vi "Append New Page.vi"(6 "Set as active (T)":bool=TRUE, 8 "error in (no error)":errorcluster, 10 "Page Name":string, 11 "Document in":refnum<class "Document.lvclass">) -> (0 "error out":errorcluster, 1 "Created?":bool, 2 "Created Page Name":string, 3 "Document out":refnum<class "Document.lvclass">)   [LabVIEW 2017, in "LabVIEW NPOI.lvlib" / "Document.lvclass"]
doc: "Create new page to the <b>Document</b>, nammed <b>Page Name</b>."
uses:
  Document.lvclass
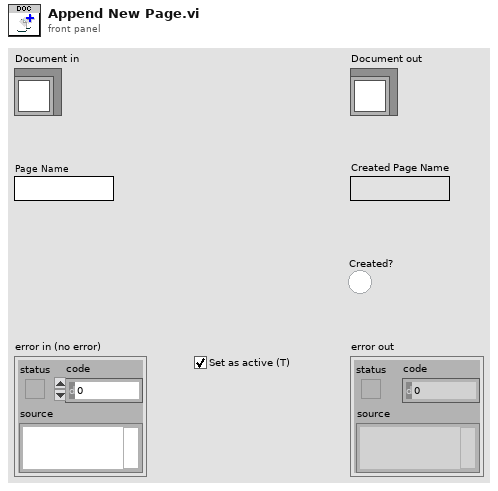
[diagram p1: front panel]
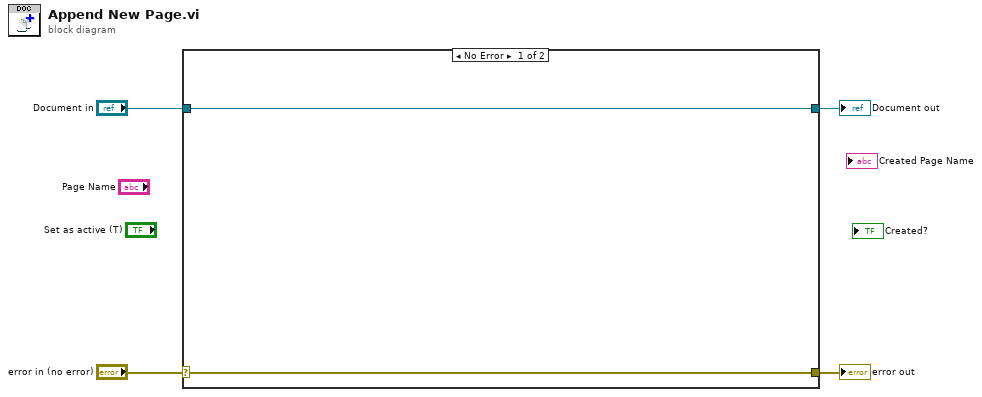
[diagram p0: block diagram]
diagram:
  n1 = case shown="No Error" "error in (no error)" {
    selector: "error in (no error)" -> [w5 w8]
    tunnel: [w5 w8] -> w3
    tunnel: [w6 w7] -> w1
    tunnel: "Document in" -> [w6 w7]
    frame No Error {
    }
    frame Error {
    }
  }
  "error out" <- w3
  "Document out" <- w1
